vi "RampScript_SingleVideo.vi"() -> ()   [LabVIEW 2017]
uses:
  FrontPanelReferences.vi
panel:
  in  "Record Time":u32=15000
  in  "B_f^2":dbl
  in  "B_0^2":dbl
  in  "Steps":i32=30
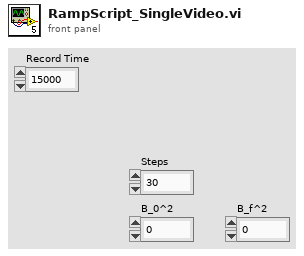
[diagram p1: front panel]
types:
  T1 = typedef "WaveformGenerator.lvlib/WaveformGeneratorInterfaceRef.ctl" = cluster{"Waveform X":refnum<vi>, "Waveform Y":refnum<vi>, "Waveform Z":refnum<vi>, "Amplitude X":refnum<vi>, "Amplitude Y":refnum<vi>, "Amplitude Z":refnum<vi>, "Frequency X":refnum<vi>, "Frequency Y":refnum<vi>, "Frequency Z":refnum<vi>, "Phase X":refnum<vi>, "Phase Y":refnum<vi>, "Phase Z":refnum<vi>, "Offset X":refnum<vi>, "Offset Y":refnum<vi>, "Offset Z":refnum<vi>, "Stop":refnum<vi>, "On/Off":refnum<vi>, "Field^2":refnum<vi>}
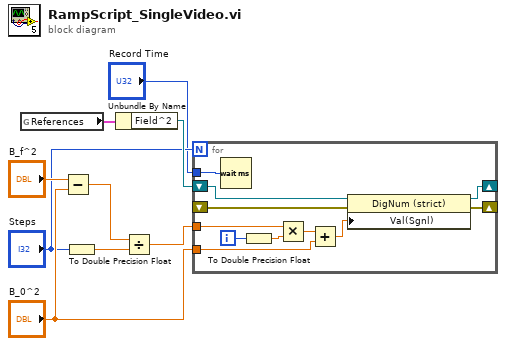
[diagram p0: block diagram]
diagram:
  n1 = global read "FrontPanelReferences.vi" "References"() -> (w9:T1)
  n2 = Subtract(x="B_f^2", y="B_0^2") -> (x-y=w3:dbl)
  n3 = To Double Precision Float(number="Steps") -> (double precision float=w4:dbl)
  n4 = Unbundle By Name(w9) -> ("Field^2"=w8:refnum<vi>)
  n5 = Divide(x=w3, y=w4) -> (x/y=w2:dbl)
  n6 = for {
    N: "Steps" -> [_]
    shift-right: [w12] -> _
    shift-left: w8 -> [w19]
    shift-right: [w11] -> _
    shift-left: _ -> [w18]
    tunnel: "B_0^2" -> [w17]
    tunnel: w2 -> [w15]
    tunnel: "Record Time" -> [w10]
    i -> [w20]
    n7 = Wait (ms)(milliseconds to wait=w10) -> ()  [unwired: 1 out]
    n8 = To Double Precision Float(number=w20) -> (double precision float=w16:dbl)
    n9 = Multiply(x=w15, y=w16) -> (x*y=w14:dbl)
    n10 = Add(x=w14, y=w17) -> (x+y=w13:dbl)
    n11 = property class="DigNum (strict)"(reference=w19, error in=w18, "Val(Sgnl)"=w13) -> (reference out=w12:refnum<vi>, error out=w11:errorcluster)
  }
